vi "Create.vi"(8 "error in (no error)":errorcluster, 10 "Comparator":refnum<class "Comparator.lvclass">) -> (0 "error out":errorcluster, 3 "One or More":refnum<class "One or More.lvclass">)   [LabVIEW 2020, in "One or More.lvlib" / "One or More.lvclass"]
uses:
  One or More.lvclass
  Core/Comparator/Comparator.lvclass
  One or More.lvclass/One or More.ctl
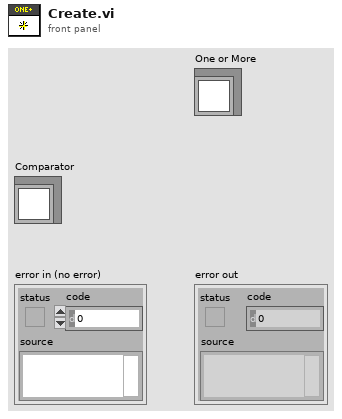
[diagram p1: front panel]
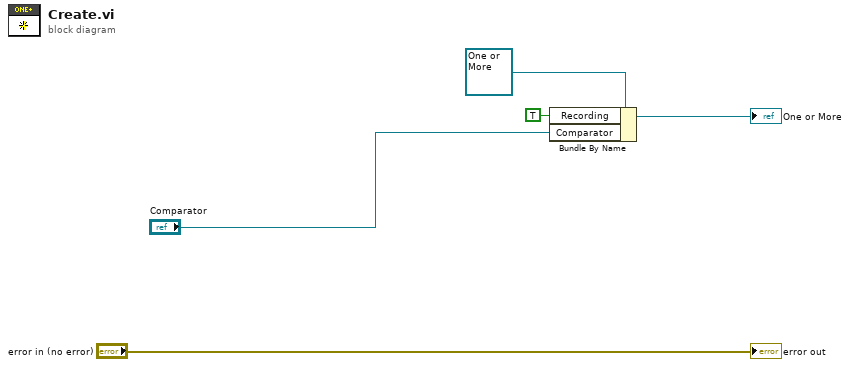
[diagram p0: block diagram]
diagram:
  n1 = Bundle By Name(cluster=refnum<class "One or More.lvclass"> refnum ("One or More"), "Recording"=TRUE, "Comparator"="Comparator") -> (→"One or More":refnum<class "One or More.lvclass">)
  "error out" <- "error in (no error)"
